vi "Recipe_to_Sequence.vi"() -> ()   [LabVIEW 2014]
uses:
  15_DataManagement/Config_RFSA_IQ_Acq.ctl
  15_DataManagement/Config_RFSA_Vertical.ctl
  15_DataManagement/Config_RFSG.ctl
  15_DataManagement/Config_RFSA_Spectrum_Acq.ctl
  <vilib>/Utility/file.llb/Read From Spreadsheet File (string).vi
panel:
  in  "file path (dialog if empty)":path=path "C:/Gyuwon_Folder/SourceCodeFolder/1005_Gyu_RF_SourceProject_Msg/___SystemFiles/RecipeVer1.ini"
  out "output cluster 3":T1 {"SG External Gain (dBm)" format="%#_6p"; "RF Power Level (dBm)" format="%#_6p"; "Carrier Frequency" format="%#_6p"}
  out "output cluster 2":T2={"Acquisition Type"=100, "Reference Level (dBm)"=0.0, "External Gain (dB)"=0.0} {"External Gain (dB)" format="%#_13g"; "Reference Level (dBm)" format="%#_13g"; "Acquisition Type" items=["IQ"=100, "Spectrum"=101]}
  out "output cluster":T3={"carrier frequency"=100000000.0, "IQ rate (S/s)"=1000000.0, "samples per record"=1000} {"IQ rate (S/s)" format="%#_6p"; "carrier frequency" format="%#_6p"}
  in  "Standard":enum16{"LTE", "WCDMA", "GSM", "EDGE", "CW"}(ring)
  out "Array":dbl[](array[numeric]) format="%#_6p"
  in  "Seq_Index":i32
  in  "DeviceSetup":variant[](array[variant])
  out "all rows":string[][](array[string])
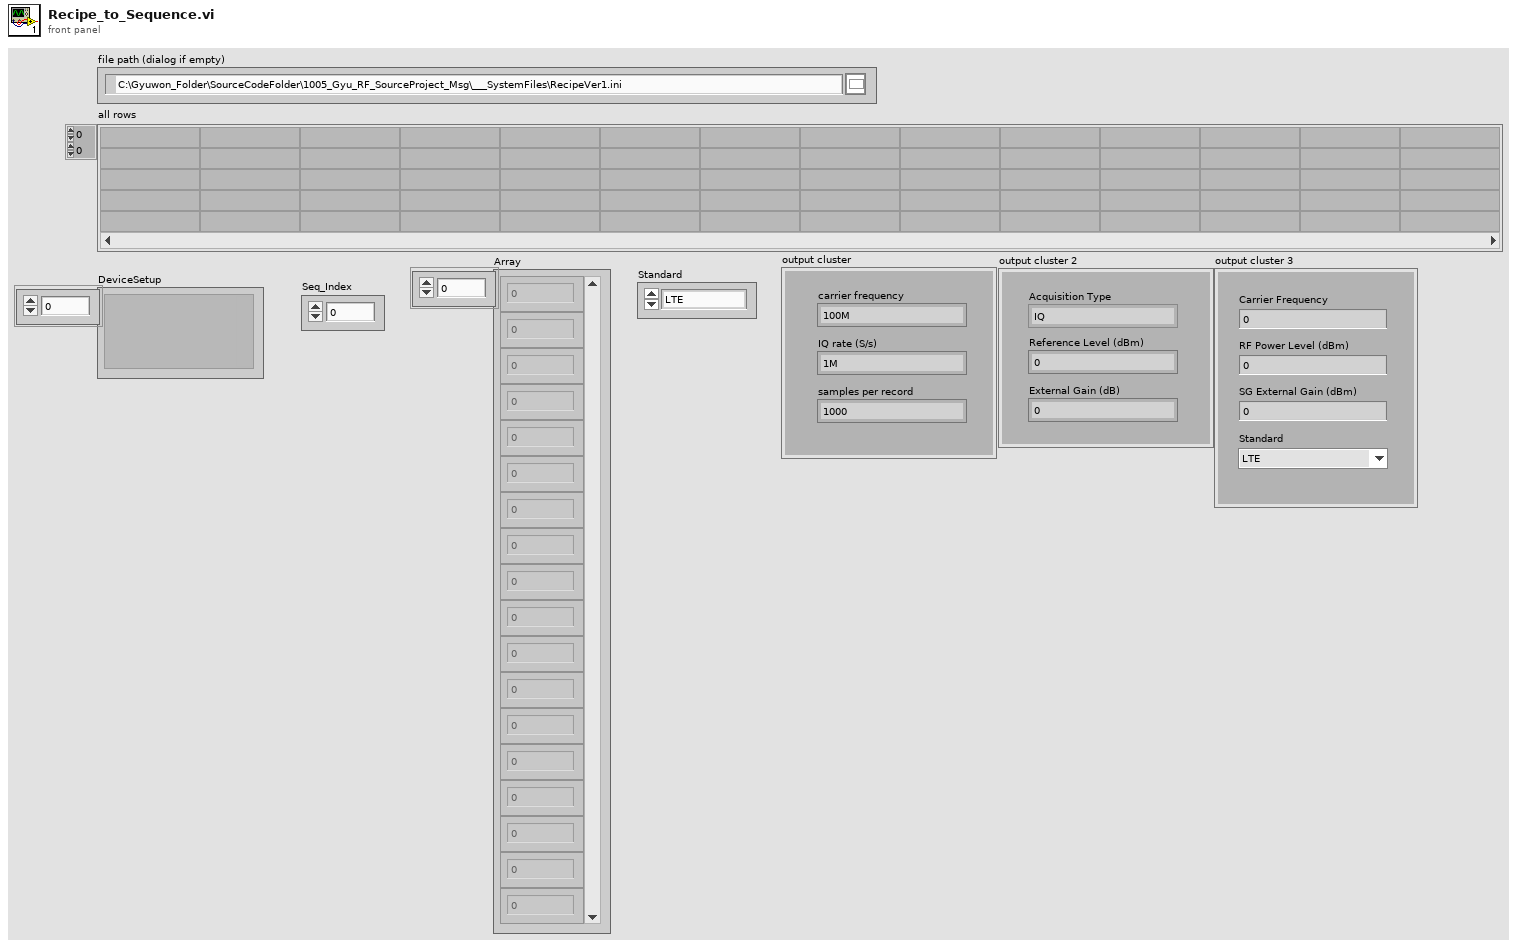
[diagram p1: front panel]
types:
  T1 = typedef "Config_RFSG.ctl" = cluster{"Carrier Frequency":dbl, "RF Power Level (dBm)":dbl, "SG External Gain (dBm)":dbl, "Standard":enum16{"LTE", "WCDMA", "GSM", "EDGE", "CW"}}
  T2 = typedef "Config_RFSA_Vertical.ctl" = cluster{"Acquisition Type":i32, "Reference Level (dBm)":dbl, "External Gain (dB)":dbl}
  T3 = typedef "Config_RFSA_IQ_Acq.ctl" = cluster{"carrier frequency":dbl, "IQ rate (S/s)":dbl, "samples per record":i64}
  T4 = typedef "Config_RFSA_Spectrum_Acq.ctl" = cluster{"Resolution Bandwidth (Hz)":dbl, "Start Frequency (Hz)":dbl, "Stop Frequency (Hz)":dbl}
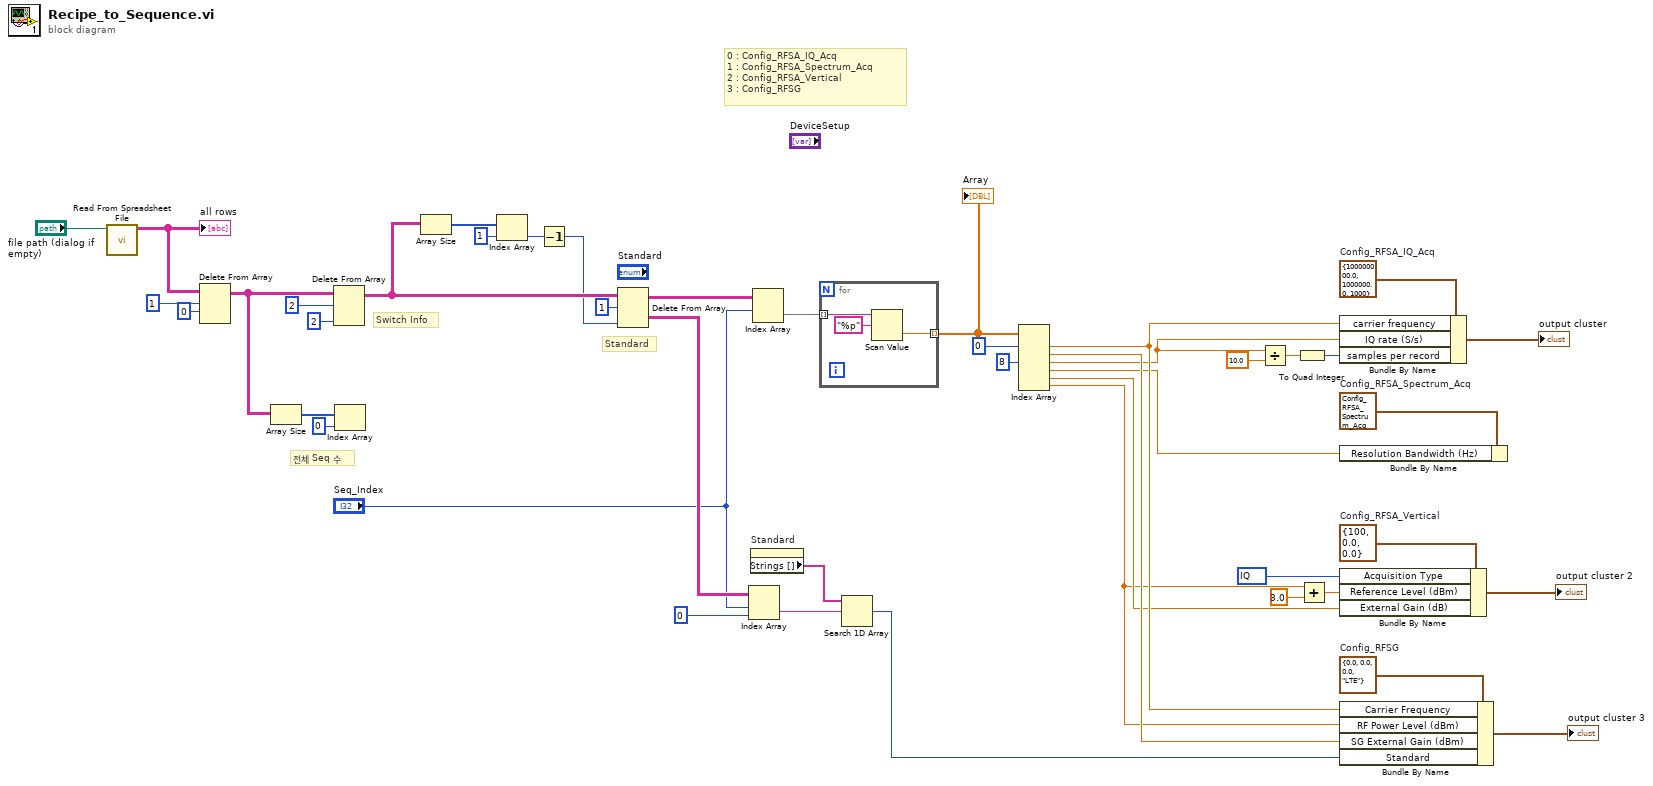
[diagram p0: block diagram]
diagram:
  w19 = 100 items=["IQ"=100, "Spectrum"=101] ("Acquisition Type")
  w24 = T3 {"carrier frequency"=100000000.0, "IQ rate (S/s)"=1000000.0, "samples per record"=1000}  # Config_RFSA_IQ_Acq
  w23 = T4 {"Resolution Bandwidth (Hz)"=10000.0, "Start Frequency (Hz)"=90000000.0, "Stop Frequency (Hz)"=110000000.0}  # Config_RFSA_Spectrum_Acq
  w22 = T2 {"Acquisition Type"=100, "Reference Level (dBm)"=0.0, "External Gain (dB)"=0.0}  # Config_RFSA_Vertical
  w25 = T1 {"Carrier Frequency"=0.0, "RF Power Level (dBm)"=0.0, "SG External Gain (dBm)"=0.0, "Standard"=enum."LTE"}  # Config_RFSG
  # "0 : Config_RFSA_IQ_Acq\n1 : Config_RFSA_Spectrum_Acq\n2 : Config_RFSA_Vertical\n3 : Config_RFSG"
  # "Switch Info"
  # "Standard"
  # "전체 Seq 수"
  n1 = call-poly <vilib>:"Read From Spreadsheet File.vi"("file path (dialog if empty)"="file path (dialog if empty)") -> ("all rows"=w44:string[][])  [unwired: 6 in, 4 out]
  "all rows" <- w44
  n2 = Delete From Array(array=w44, length=1, index (row)=0) -> (array with subset deleted=w39:string[][])  [unwired: 1 in, 1 out]
  n3 = Array Size(array=w39) -> (size(s)=w41:i32[])
  n4 = Delete From Array(array=w39, length=2, index (col)=2 ("disabled index (col)")) -> (array with subset deleted=w34:string[][])  [unwired: 1 in, 1 out]
  n5 = Index Array(array=w41, index=0) -> ()  [unwired: 1 out]
  n6 = Array Size(array=w34) -> (size(s)=w36:i32[])
  n7 = Index Array(array=w36, index=1) -> (element=w33:i32)
  n8 = Decrement(x=w33) -> (x-1=w31:i32)
  n9 = Delete From Array(array=w34, length=1, index (col)=w31) -> (deleted portion=w9:string[][], array with subset deleted=w30:string[][])  [unwired: 1 in]
  n10 = Index Array(array=w9, index (row)="Seq_Index", index (col)=0 ("disabled index (col)")) -> (element=w6:string)
  n11 = property on="Standard" class="Enum (strict)"() -> ("Strings []"=w5:string[])  [unwired: 2 in, 2 out]
  n12 = Index Array(array=w30, index (row)="Seq_Index") -> (element=w29:string[])  [unwired: 1 in]
  n13 = for {
    tunnel: w29 -> [w48] mode=indexing
    tunnel: [w46] -> w28 mode=indexing
    n14 = Scan Value(string=w48, format string="%p") -> (value=w46:dbl)  [unwired: 1 in, 1 out]
  }
  "Array" <- w28
  n15 = Search 1D Array(1D array=w5, element=w6) -> (index of element=w4:i32)  [unwired: 1 in]
  n16 = Index Array(array=w28, index #1=0 ("index"), index #3=8 ("index")) -> (element #1=w26:dbl, element #2=w21:dbl, element #3=w11:dbl, element #4=w18:dbl, element #5=w17:dbl, element #6=w15:dbl)  [unwired: 4 in]
  n17 = Divide(x=w11, y=10.0) -> (x/y=w13:dbl)
  n18 = To Quad Integer(1:w13) -> (0:w12:i64)
  n19 = Add(x=w15, y=3.0) -> (x+y=w16:dbl)
  n20 = Bundle By Name(cluster=w24, "carrier frequency"=w26, "IQ rate (S/s)"=w11, "samples per record"=w12) -> (→"output cluster":T3)
  n21 = Bundle By Name(cluster=w23, "Resolution Bandwidth (Hz)"=w18) -> ()  [unwired: 1 out]
  n22 = Bundle By Name(cluster=w22, "Acquisition Type"=w19, "Reference Level (dBm)"=w16, "External Gain (dB)"=w17) -> (→"output cluster 2":T2)
  n23 = Bundle By Name(cluster=w25, "Carrier Frequency"=w26, "RF Power Level (dBm)"=w15, "SG External Gain (dBm)"=w21, "Standard"=w4) -> (→"output cluster 3":T1)
